vi "bpm.vi"() -> ()   [LabVIEW 2016, in "features.lvlib"]
doc: "The bpm vi uses the source rio to control the bpms on the high voltage deck. It can only work if the source rio is in the same project as this vi."
uses:
  Features/features/features.lvlib
panel:
  in  "error in (no error)":errorcluster
  out "error out":errorcluster
  in  "stop":bool
  in  "Source 2 X10":bool
  in  "Source 2 BPM":bool
  in  "Source 1 X 10":bool
  in  "Source 1 BPM":bool
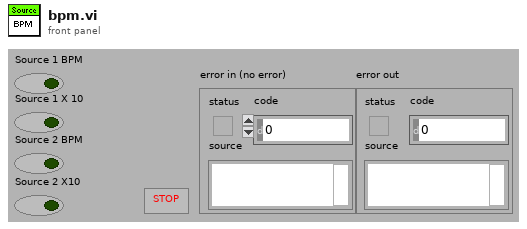
[diagram p1: front panel]
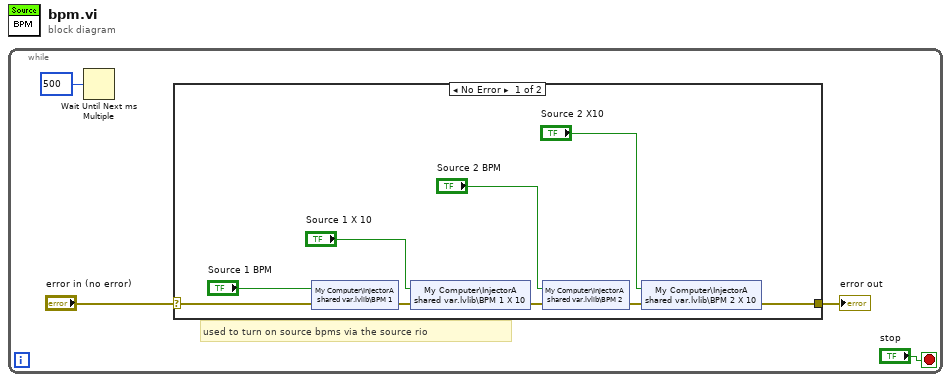
[diagram p0: block diagram]
diagram:
  n1 = while {
    stop <- "stop" stop-if-true
    # "used to turn on source bpms via the source rio"
    n2 = Wait Until Next ms Multiple(millisecond multiple=u32 500) -> ()  [unwired: 1 out]
    n3 = case shown="No Error" "error in (no error)" {
      selector: "error in (no error)" -> [w5 w14]
      tunnel: [w6 w14] -> w2
      frame No Error {
        n4 = shared-variable "My Computer\\InjectorA shared var.lvlib\\BPM 1"("Source 1 BPM", error in=w5) -> (error out=w9:errorcluster)
        n5 = shared-variable "My Computer\\InjectorA shared var.lvlib\\BPM 1 X 10"("Source 1 X 10", error in=w9) -> (error out=w8:errorcluster)
        n6 = shared-variable "My Computer\\InjectorA shared var.lvlib\\BPM 2"("Source 2 BPM", error in=w8) -> (error out=w7:errorcluster)
        n7 = shared-variable "My Computer\\InjectorA shared var.lvlib\\BPM 2 X 10"("Source 2 X10", error in=w7) -> (error out=w6:errorcluster)
      }
      frame Error {
      }
    }
    "error out" <- w2
  }
